vi "Yokogawa WT1800 Series Measure Harmonics.vi"() -> ()   [LabVIEW 2015]
doc: "This example shows how to measure the harmonic measurement numeric list data.\n\n<b>Note:</b>\nThis setting valid on models with the harmonic measurement (/G5 or /G6) option."
uses:
  <instrlib>/Yokogawa WT1800 Series/Public/Data/Low Level/Fetch Measurement (Harmonics).vi
  <instrlib>/Yokogawa WT1800 Series/Yokogawa WT1800 Series.lvlib
panel:
  in  "Function (1: U)":i32(ring)=1 items=["U"=1, "I"=2, "P"=3, "S"=4, "Q"=5, "Lambda"=6, "Phi"=7, "Phi U"=8, "Phi I"=9, "Z"=10, "Rs"=11, "Xs"=12, "Rp"=13, "Xp"=14, "UHDF"=15, "IHDF"=16, "PHDF"=17]
  in  "Max Order (0: All)":i32 min=0 max=500
  out "Measurement":dbl[](array[numeric])
  out "Function":string
  in  "Item (1)":i32=1 min=1 max=64 step=1
  in  "Element (1: 1)":i32(ring)=1 items=["1"=1, "2"=2, "3"=3, "4"=4, "5"=5, "6"=6, "Sigma A"=7, "Sigma B"=8, "Sigma C"=9]
  in  "Timeout (10000 ms)":i32=10000 min=1
  in  "VISA resource name":refnum<visa-resource-name>
  # "(c) 2011 Yokogawa Meters & Instruments Corporation.  All rights reserved."
  # "WT1800 SERIES POWER ANALYZER"
  # "Total        DC            1             2              3             4"
  # "ms"
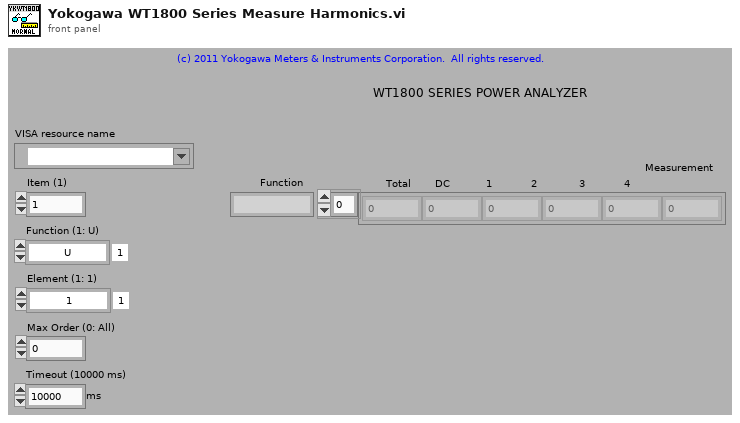
[diagram p1: front panel]
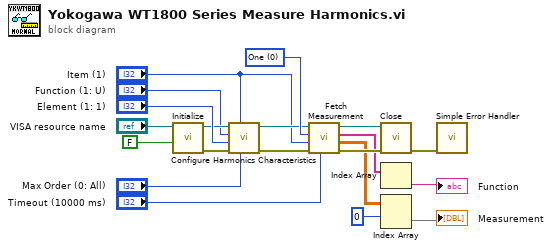
[diagram p0: block diagram]
diagram:
  w15 = 0 items=["One", "Plural"] ("Measure Item (1: Plural)")
  n1 = call <instrlib>:"Initialize.vi"("Reset (True)"=FALSE ("Reset? (True)"), "VISA resource name"="VISA resource name") -> ("error out"=w4:errorcluster, "VISA resource name out"=w5:refnum<visa-resource-name>)  [unwired: 8 in]
  n2 = call <instrlib>:"Configure Harmonics Characteristics.vi"("Max Order (0: All)"="Max Order (0: All)", "Item (1)"="Item (1)", "error in (no error)"=w4, "Element/Wiring Unit (1: 1)"="Element (1: 1)", "Function (0: None)"="Function (1: U)", "VISA resource name"=w5) -> ("error out"=w13:errorcluster, "VISA resource name out"=w14:refnum<visa-resource-name>)  [unwired: 4 in]
  n3 = call-poly <instrlib>:"Fetch Measurement.vi"("Timeout (10000 ms)"="Timeout (10000 ms)", "error in (no error)"=w13, "Number of Item (15)"="Item (1)", "Measure Item (1: Plural)"=w15, "VISA resource name"=w14) -> ("error out"=w17:errorcluster, "Measurement"=w12:dbl[][], "Function"=w9:string[], "VISA resource name out"=w18:refnum<visa-resource-name>)  [unwired: 3 in]
  n4 = call <instrlib>:"Close.vi"("error in (no error)"=w17, "VISA resource name"=w18) -> ("error out"=w20:errorcluster)  [unwired: 9 in]
  n5 = Index Array(array=w9) -> (element=→"Function":string)  [unwired: 1 in]
  n6 = Index Array(array=w12, index (row)=0 ("指標 （行）")) -> (element=→"Measurement":dbl[])  [unwired: 1 in]
  n7 = call <vilib>:"Simple Error Handler.vi"("error in (no error)"=w20) -> ()  [unwired: 4 in, 5 out]
